vi "Next Post Processor Name.vi"(7 "Ack Result":refnum<class "Acquired Result.lvclass">, 8 "error in (no error)":errorcluster, 11 "Monitor-Pulse in":refnum<class "Application Controller.lvclass">) -> (0 "error out":errorcluster, 1 "Complete":bool, 2 "Post processor name":string, 3 "Monitor-Pulse out":refnum<class "Application Controller.lvclass">, 5 "Ack Result out":refnum<class "Acquired Result.lvclass">)   [LabVIEW 2018, in "Application Controller.lvclass"]
uses:
  Application Controller.lvclass
  NHMFL_Core/Libraries/Instruments/Results/Acquired Result/Acquired Result.lvclass
  Application Controller.lvclass/Application Controller.ctl
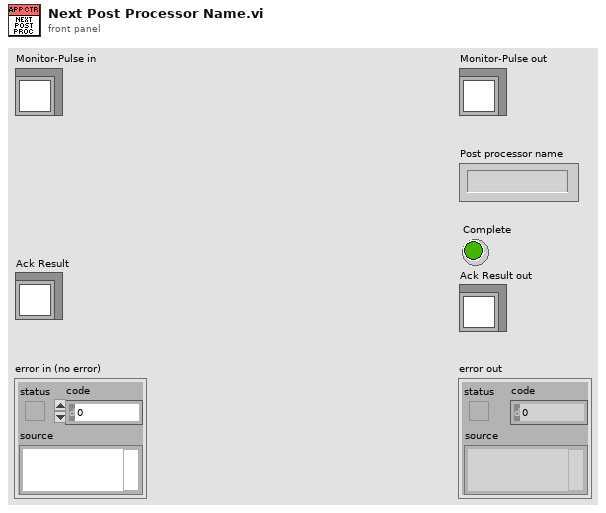
[diagram p1: front panel]
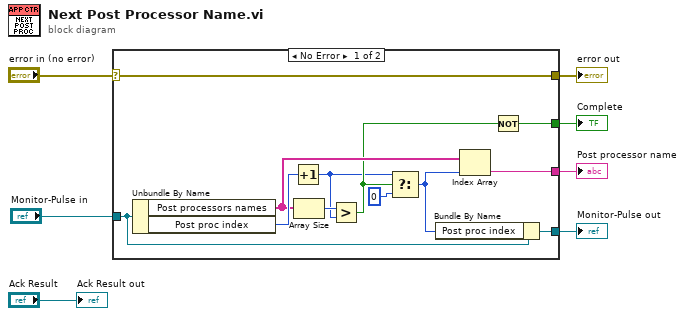
[diagram p0: block diagram]
diagram:
  n1 = case shown="No Error" "error in (no error)" {
    selector: "error in (no error)" -> [w19 w21]
    tunnel: [w19 w21] -> w6
    tunnel: [w14 w20] -> w4
    tunnel: "Monitor-Pulse in" -> [w18 w20]
    tunnel: [w16 _] -> w3
    tunnel: [w9 _] -> w2
    frame No Error {
      n2 = Unbundle By Name(w18) -> ("Post processors names"=w15:string[], "Post proc index"=w17:i32)
      n3 = Increment(x=w17) -> (x+1=w8:i32)
      n4 = Array Size(array=w15) -> (size(s)=w13:i32)
      n5 = Greater?(x=w13, y=w8) -> (0:w12:bool)
      n6 = Select(t=w8, s=w12, f=0 ("t")) -> (s? t:f=w10:i32)
      n7 = Bundle By Name(cluster=w18, "Post proc index"=w10) -> (w14:refnum<class "Application Controller.lvclass">)
      n8 = Index Array(array=w15, index=w10) -> (element=w16:string)
      n9 = Not(x=w12) -> (.not. x?=w9:bool)
    }
    frame Error {
    }
  }
  "error out" <- w6
  "Monitor-Pulse out" <- w4
  "Complete" <- w2
  "Post processor name" <- w3
  "Ack Result out" <- "Ack Result"
